vi "Test all.vi"() -> ()   [LabVIEW 2018]
uses:
  <vilib>/addons/_JKI Toolkits/Caraya/classes/Test/Test.lvclass
panel:
  out "error out":errorcluster
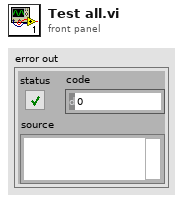
[diagram p1: front panel]
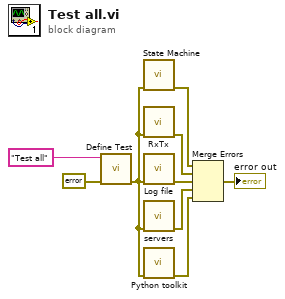
[diagram p0: block diagram]
diagram:
  n1 = call <vilib>:"Define Test.vi"("error in (no error)"=errorcluster {"status"=FALSE, "code"=0, "source"=""}, "Label (VI Title)"="Test all") -> ("error out"=w2:errorcluster)  [unwired: 8 in, 1 out]
  n2 = call "State Machine.vi"("error in (no error)"=w2) -> ("error out"=w7:errorcluster)  [unwired: 10 in]
  n3 = call "RxTx.vi"("error in (no error)"=w2) -> ("error out"=w6:errorcluster)  [unwired: 10 in]
  n4 = call "Log file.vi"("error in (no error)"=w2) -> ("error in (no error) 2"=w4:errorcluster)  [unwired: 10 in]
  n5 = call "servers.vi"("error in (no error)"=w2) -> ("error out"=w3:errorcluster)  [unwired: 10 in]
  n6 = call "Python toolkit.vi"("error in (no error)"=w2) -> ("error out"=w1:errorcluster)  [unwired: 10 in]
  n7 = Merge Errors(w7, w6, w4, w3, w1) -> (→"error out":errorcluster)
